vi "AreaTriangle.vi"() -> ()   [LabVIEW 2023]
panel:
  in  "stop":bool
  out "Area (cm^2)":dbl
  in  "Height (cm)":dbl
  in  "Base (cm)":dbl
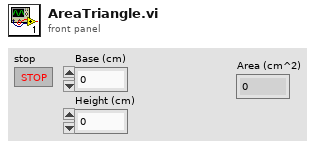
[diagram p1: front panel]
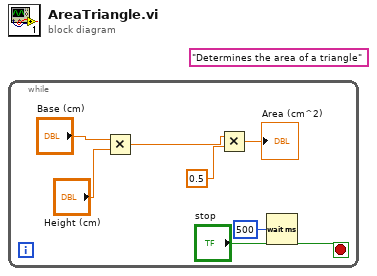
[diagram p0: block diagram]
diagram:
  (unwired) "Determines the area of a triangle"
  n1 = while {
    stop <- "stop" stop-if-true
    n2 = Multiply(x="Base (cm)", y="Height (cm)") -> (x*y=w5:dbl)
    n3 = Multiply(x=w5, y=0.5) -> (x*y=→"Area (cm^2)":dbl)
    n4 = Wait (ms)(milliseconds to wait=u32 500) -> ()  [unwired: 1 out]
  }
